vi "Build Array (Multi).vi"(8 "error in (no error)":errorcluster, 10 "JSON Datatypes":refnum<class "JSON Datatype.lvclass">[](array[class]), 11 "JSON Array in":refnum<class "JSON Array.lvclass">) -> (0 "error out":errorcluster, 3 "JSON Array out":refnum<class "JSON Array.lvclass">)   [LabVIEW 2017, in "LVJSON.lvlib" / "JSON Array.lvclass"]
uses:
  JSON Array.lvclass
  JSON Datatype/JSON Datatype.lvclass
  JSON Array.lvclass/JSON Array.ctl
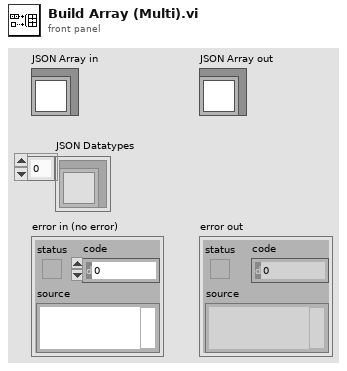
[diagram p1: front panel]
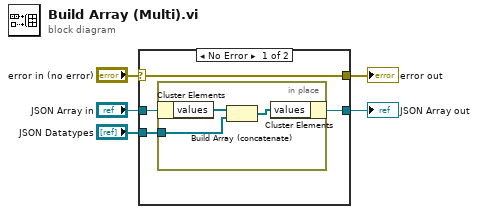
[diagram p0: block diagram]
diagram:
  n1 = case shown="No Error" "error in (no error)" {
    selector: "error in (no error)" -> [w6 w14]
    tunnel: [w6 w14] -> w4
    tunnel: [w7 w13] -> w2
    tunnel: "JSON Array in" -> [w9 w13]
    tunnel: "JSON Datatypes" -> [w8 _]
    frame No Error {
      n2 = in-place {
        in-place-border: w8 -> [w11]
        n3 = in-place-cluster #1(w9) -> ("values"=w12:refnum<class "JSON Datatype.lvclass">[])
        n4 = Build Array (concatenate)(w12, w11) -> (w10:refnum<class "JSON Datatype.lvclass">[])
        n5 = in-place-cluster #1("values"=w10) -> (w7:refnum<class "JSON Array.lvclass">)
      }
    }
    frame Error {
    }
  }
  "error out" <- w4
  "JSON Array out" <- w2
